vi "OnDataChange.vi"(0 "GRMActor in":refnum<class "GenericActor.lvclass">, 1 "DataExchange":T1, 3 "error in (no error)":errorcluster) -> (7 "GRMActor out":refnum<class "GenericActor.lvclass">, 10 "error out":errorcluster)   [LabVIEW 2020, in "GenericActor.lvlib" / "GenericActor.lvclass"]
uses:
  GenericActor.lvclass
  Device/Device/DataExchange.ctl
  <vilib>/ActorFramework/Message Enqueuer/Message Priority.ctl
  Interface/DataListener Messages/OnDataChange Msg/OnDataChange Msg.lvclass/OnDataChange Msg.ctl
  <vilib>/ActorFramework/Message Enqueuer/Message Enqueuer.lvclass/Message Enqueuer.ctl
  <vilib>/ActorFramework/Message Enqueuer/Message Enqueuer.lvclass
  GenericActor.lvclass/GenericActor.ctl
  <vilib>/ActorFramework/Message Enqueuer/Enqueue.vi
  Interface/DataListener Messages/OnDataChange Msg/OnDataChange Msg.lvclass
  C:/Program Files/National Instruments/LabVIEW 2020/vi.lib/ActorFramework/Message/Message.lvclass
  <vilib>/ActorFramework/Message Priority Queue/Priority Enqueue.vi
  Interface/DataListener/DataListener.lvclass
panel:
  out "error out 2":errorcluster
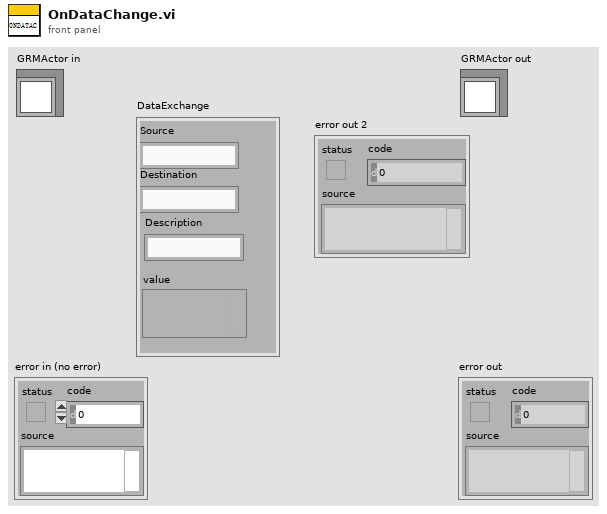
[diagram p1: front panel]
types:
  T1 = typedef "DataListener.lvclass/DataExchange.ctl" = cluster{"Source":string, "Destination":string, "Description":string, "value":variant}
  T2 = typedef "Actor Framework.lvlib/Message Enqueuer.lvclass/Message Priority.ctl" = enum16{"Low", "Normal", "High"}
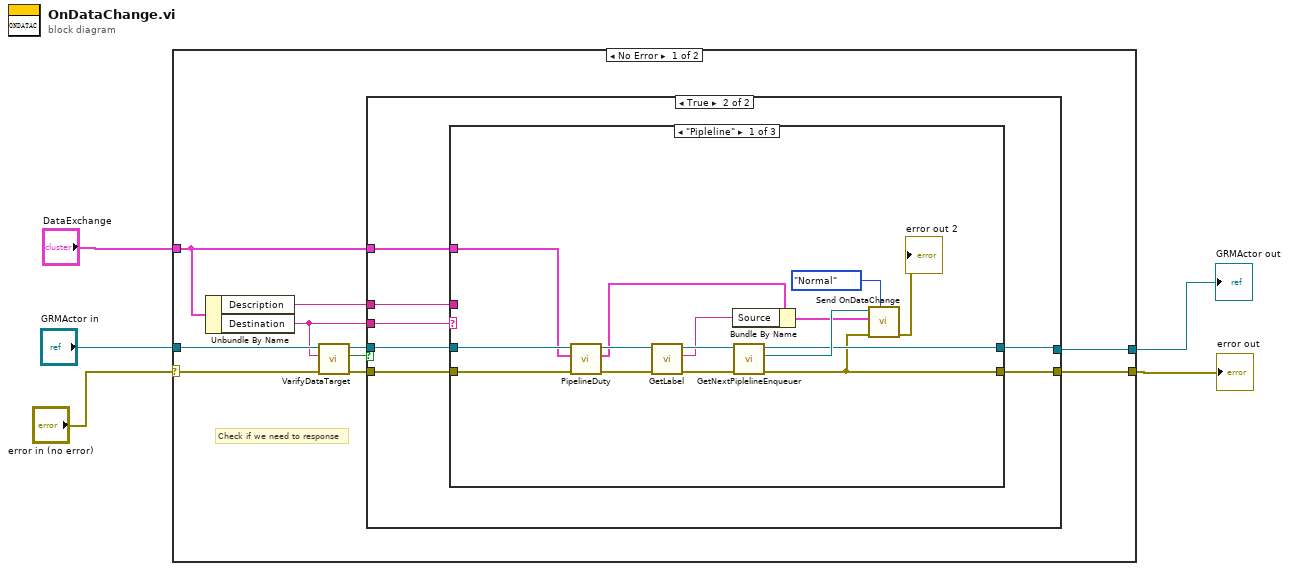
[diagram p0: block diagram]
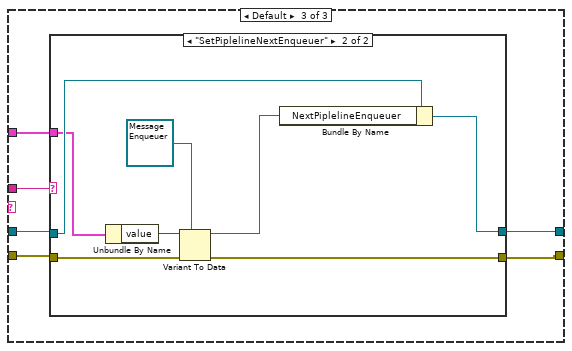
[diagram p4: hidden frame]
diagram:
  n1 = case shown="No Error" "error in (no error)" {
    selector: "error in (no error)" -> [w13 w59]
    tunnel: [w14 w59] -> w4
    tunnel: "GRMActor in" -> [w11 w58]
    tunnel: [w15 w58] -> w3
    tunnel: "DataExchange" -> [w9 _]
    frame No Error {
      # "Check if we need to response"
      n2 = Unbundle By Name(w9) -> ("Description"=w7:string, "Destination"=w6:string)
      n3 = call-dynamic "VarifyDataTarget.vi"("error in (no error)"=w13, "Destination"=w6, "GRMActor in"=w11) -> ("error out"=w12:errorcluster, "Response?"=w8:bool, "GRMActor out"=w10:refnum<class "GenericActor.lvclass">)  [unwired: 6 in]
      n4 = case shown="True" w8 {
        tunnel: [w17 w24] -> w15
        tunnel: w10 -> [w17 w23]
        tunnel: [w16 w21] -> w14
        tunnel: w12 -> [w16 w22]
        tunnel: w9 -> [_ w20]
        tunnel: w7 -> [_ w19]
        tunnel: w6 -> [_ w18]
        frame False {
        }
        frame True {
          n5 = case shown="\"Pipleline\"" w18 {
            tunnel: [w28 w40 w47] -> w24
            tunnel: w23 -> [w30 w40 w46]
            tunnel: w22 -> [w31 w41 w45]
            tunnel: [w27 w41 w44] -> w21
            tunnel: w20 -> [w29 _ w43]
            tunnel: w19 -> [_ _ w42]
            frame "Pipleline" {
              n6 = call-dynamic "PipelineDuty.vi"("error in (no error)"=w31, "DataExchange"=w29, "GRMActor in"=w30) -> ("error out"=w39:errorcluster, "DataExchange 2"=w33:T1, "GRMActor out"=w37:refnum<class "GenericActor.lvclass">)  [unwired: 6 in]
              n7 = call-dynamic "GetLabel.vi"("error in (no error)"=w39, "GRMActor in"=w37) -> ("error out"=w38:errorcluster, "Label"=w32:string, "GRMActor out"=w36:refnum<class "GenericActor.lvclass">)  [unwired: 7 in]
              n8 = Bundle By Name(cluster=w33, "Source"=w32) -> (w34:T1)
              n9 = call-dynamic "GetNextPiplelineEnqueuer.vi"("error in (no error)"=w38, "GRMActor in"=w36) -> ("error out"=w27:errorcluster, "NextPiplelineEnqueuer"=w35:refnum<class "Message Enqueuer.lvclass">, "GRMActor out"=w28:refnum<class "GenericActor.lvclass">)  [unwired: 7 in]
              n10 = call "Send OnDataChange.vi"("Message Priority (Normal)"=Message_Priority."Normal", "error in (no error)"=w27, "DataExchange"=w34, "Message Enqueuer"=w35) -> ("error out"=→"error out 2":errorcluster)  [unwired: 6 in, 1 out]
            }
            frame "Broadcast" {
            }
            frame Default {
              n11 = case shown="\"SetPiplelineNextEnqueuer\"" w42 {
                tunnel: [w49 w54] -> w47
                tunnel: w46 -> [w49 w55]
                tunnel: [w48 w56] -> w44
                tunnel: w45 -> [w48 w57]
                tunnel: w43 -> [_ w53]
                frame Default {
                }
                frame "SetPiplelineNextEnqueuer" {
                  n12 = Unbundle By Name(w53) -> ("value"=w52:variant)
                  n13 = Variant To Data(error in=w57, type=refnum<class "Message Enqueuer.lvclass"> refnum ("Enqueuer"), Variant=w52) -> (data=w50:refnum<class "Message Enqueuer.lvclass">, error out=w56:errorcluster)
                  n14 = Bundle By Name(cluster=w55, "NextPiplelineEnqueuer"=w50) -> (w54:refnum<class "GenericActor.lvclass">)
                }
              }
            }
          }
        }
      }
    }
    frame Error {
    }
  }
  "error out" <- w4
  "GRMActor out" <- w3
